vi "Write Enumerated Resources.vi"(8 "error in (no error)":errorcluster, 10 "Enumerated Resources":T1[](array[typedef]), 11 "AbstractResourceEnumerator in":refnum<class "AbstractResourceEnumerator.lvclass">) -> (0 "error out":errorcluster, 3 "AbstractResourceEnumerator out":refnum<class "AbstractResourceEnumerator.lvclass">)   [LabVIEW 2023, in "HAF.lvlib" / "AbstractResourceEnumerator.lvclass"]
doc: "Saves a new collection of Resources attached to the system."
uses:
  AbstractResourceEnumerator.lvclass
  AbstractResourceEnumerator.lvclass/AbstractResourceEnumerator.ctl
  Resource Structure.ctl
  HAF.lvlib
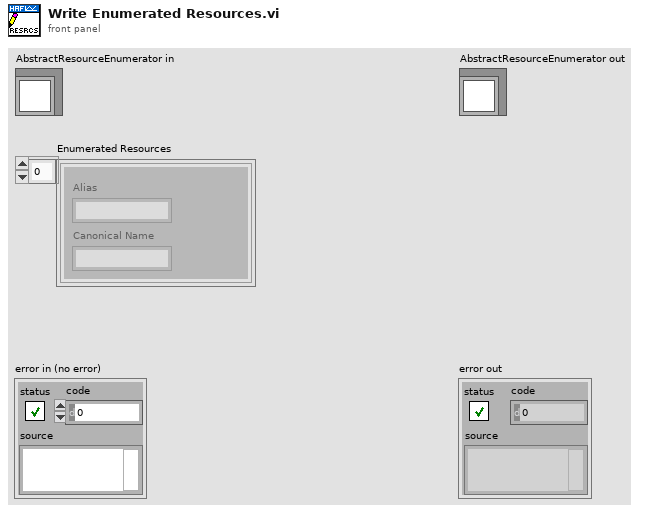
[diagram p1: front panel]
types:
  T1 = typedef "HAF.lvlib/Resource Structure.ctl" = cluster{"Alias":string, "Canonical Name":string}
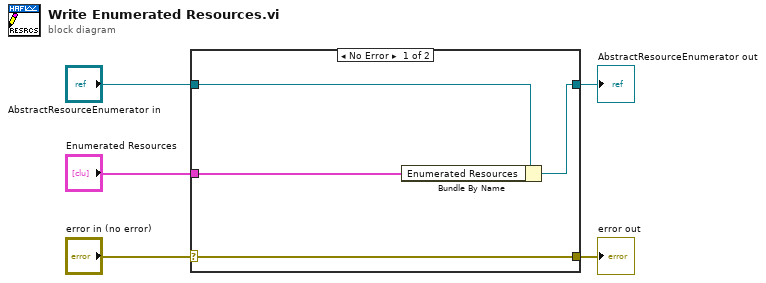
[diagram p0: block diagram]
diagram:
  n1 = case shown="No Error" "error in (no error)" {
    selector: "error in (no error)" -> [w9 w10]
    tunnel: [w9 w10] -> w4
    tunnel: [w7 w11] -> w2
    tunnel: "AbstractResourceEnumerator in" -> [w8 w11]
    tunnel: "Enumerated Resources" -> [w6 _]
    frame No Error {
      n2 = Bundle By Name(cluster=w8, "Enumerated Resources"=w6) -> (w7:refnum<class "AbstractResourceEnumerator.lvclass">)
    }
    frame Error {
    }
  }
  "error out" <- w4
  "AbstractResourceEnumerator out" <- w2
